vi "DAQmx Create Channel (AI-Force-Bridge-Polynomial).vi"(0 "task in":refnum<k21>, 1 "maximum value":dbl=100.0 format="%0.2f", 2 "minimum value":dbl=-100.0 format="%0.2f", 3 "bridge information":T1={"bridge configuration"=10182, "voltage excitation source"=10200, "voltage excitation value"=2.5, "nominal bridge resistance"=350.0} {"voltage excitation source" items=["Internal"=10200, "External"=10167]; "bridge configuration" items=["Full Bridge"=10182, "Half Bridge"=10187, "Quarter Bridge"=10270]}, 5 "physical channels":tag, 7 "name to assign":string, 9 "units":i32(ring)=15876 items=["Newtons"=15875, "Pounds"=15876, "kgf"=15877, "From Custom Scale"=10065], 11 "error in":errorcluster, 12 "custom scale name":tag, 14 "scaling information":T2={"forward coeff"=[0.0, 50.0], "reverse coeff"=[0.0, 0.02], "electrical units"=15897, "physical units"=15876} {"electrical units" items=["Volts/Volt"=15896, "mVolts/Volt"=15897]; "physical units" items=["Newtons"=15875, "Pounds"=15876, "kgf"=15877]}) -> (4 "task out":refnum<k21>, 15 "error out":errorcluster)   [LabVIEW 2020]
doc: "Creates channel(s) that use a Wheatstone bridge to measure force or load. Use this instance with sensors whose specifications provide a polynomial to convert electrical values to physical values. When you use this scaling type, NI-DAQmx requires coefficients for a polynomial that converts electrical values to physical values (forward), as well as coefficients for a polynomial that converts physical values to electrical values (reverse). If you only know one set of coefficients, use the DAQmx Compute Reverse Polynomial Coefficients VI to generate the other set."
uses:
  nilvaiu.dll
panel:
  # "input limits"
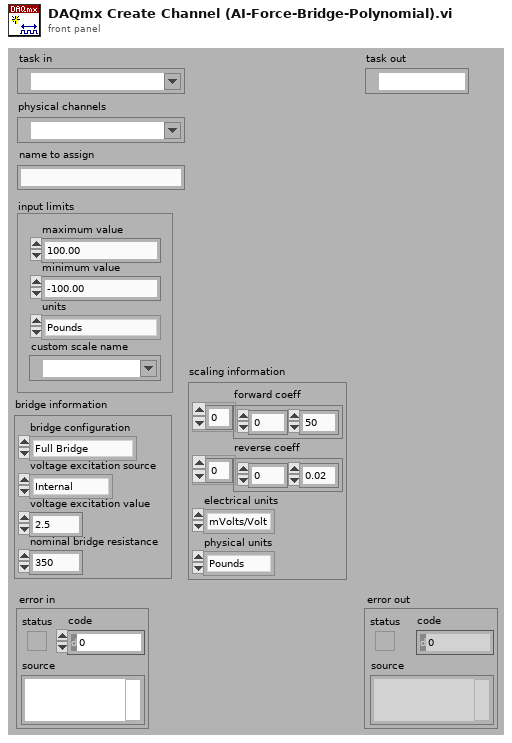
[diagram p1: front panel]
types:
  T1 = cluster{"bridge configuration":i32, "voltage excitation source":i32, "voltage excitation value":dbl, "nominal bridge resistance":dbl}
  T2 = cluster{"forward coeff":dbl[], "reverse coeff":dbl[], "electrical units":i32, "physical units":i32}
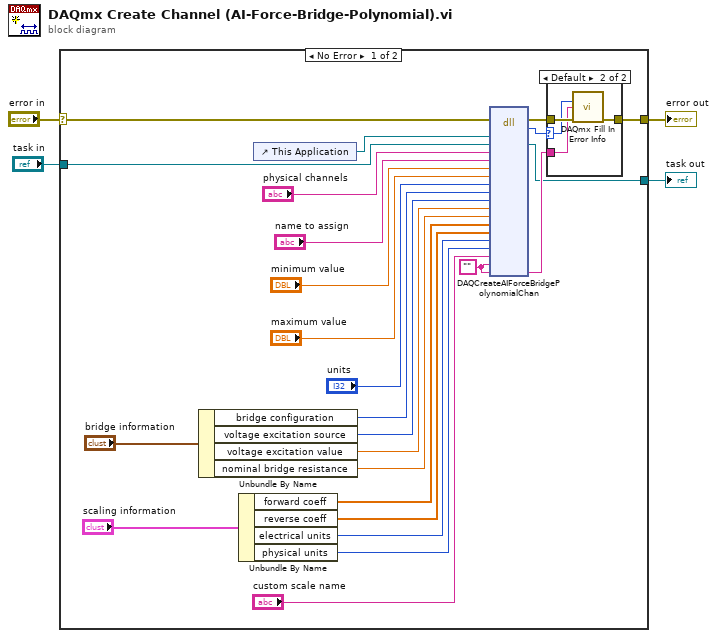
[diagram p0: block diagram]
diagram:
  n1 = case shown="No Error" "error in" {
    selector: "error in" -> [w20 w35]
    tunnel: [w27 w35] -> w4
    tunnel: "task in" -> [w21 w36]
    tunnel: [w6 w36] -> w1
    frame No Error {
      w5 = ""
      n2 = Unbundle By Name("bridge information") -> ("bridge configuration"=w11:i32, "voltage excitation source"=w10:i32, "voltage excitation value"=w9:dbl, "nominal bridge resistance"=w8:dbl)
      n3 = Unbundle By Name("scaling information") -> ("forward coeff"=w15:dbl[], "reverse coeff"=w14:dbl[], "electrical units"=w13:i32, "physical units"=w12:i32)
      n4 = control-ref of="This Application"() -> (w24:refnum<vi>)
      n5 = dll-call lib="nilvaiu.*" fn="DAQCreateAIForceBridgePolynomialChan"(error in=w20, "lvAppRef"=w24, "refObjPtr"=w21, "physicalChannelName"="physical channels", "channelNameIn"="name to assign", "minVal"="minimum value", "maxVal"="maximum value", "units"="units", "bridgeConfig"=w11, "voltageExcitSource"=w10, "voltageExcitVal"=w9, "nominalBridgeResistance"=w8, "forwardCoeffs"=w15, "reverseCoeffs"=w14, "electricalUnits"=w13, "physicalUnits"=w12, "customScaleName"="custom scale name", "channelNamesOut"=w5, "extenedErrorInfo"=w5) -> (error out=w25:errorcluster, "return type"=w7:i32, "refObjPtr"=w6:refnum<k21>, "extenedErrorInfo"=w26:string)  [unwired: 18 in, 1 out]
      n6 = case shown="Default" w7 {
        selector: w7 -> [_ w32]
        tunnel: w25 -> [w30 w34]
        tunnel: [w30 w33] -> w27
        tunnel: w26 -> [_ w31]
        frame 0 {
        }
        frame Default {
          n7 = call "DAQmx Fill In Error Info.vi"("status code"=w32, "extended error info"=w31, "error in"=w34) -> ("error out"=w33:errorcluster)  [unwired: 1 in, 11 out]
        }
      }
    }
    frame Error {
    }
  }
  "error out" <- w4
  "task out" <- w1
